vi "原始记录路径.vi"(9 "目标温度":string(combo), 11 "文件夹名称":string) -> (1 "file exists?":bool caption="文件或文件夹存在？", 3 "保存路径":path)   [LabVIEW 2015]
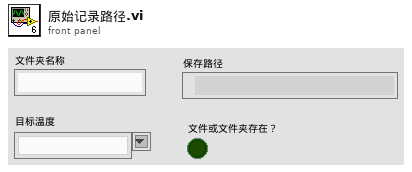
[diagram p1: front panel]
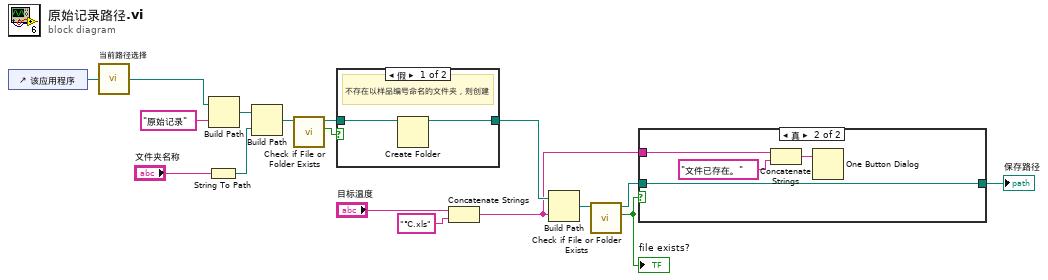
[diagram p0: block diagram]
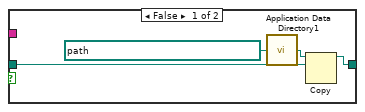
[diagram p2: hidden frame]
diagram:
  n1 = control-ref of="该应用程序"() -> (w17:refnum<vi>)
  n2 = call "当前路径选择.vi"("本应用程序"=w17) -> ("当前路径"=w16:path)
  n3 = String To Path(string="文件夹名称") -> (path=w1:path)
  n4 = Build Path(base path=w16, name or relative path="原始记录" ("名称或相对路径")) -> (appended path=w14:path)
  n5 = Build Path(base path=w14, name or relative path=w1) -> (appended path=w13:path)
  n6 = call <vilib>:"Check if File or Folder Exists.vi"("path"=w13) -> ("file or folder exists?"=w12:bool, "dup path"=w11:path)  [unwired: 8 in, 1 out]
  n7 = case shown="假" w12 {
    tunnel: w11 -> [w19 w20]
    tunnel: [w18 w20] -> w8
    frame False {
      # "不存在以样品编号命名的文件夹，则创建"
      n8 = Create Folder(path (use dialog)=w19) -> (created path=w18:path)  [unwired: 2 in, 2 out]
    }
    frame True {
    }
  }
  n9 = Concatenate Strings("目标温度", "℃.xls" ("字符串")) -> (w5:string)
  n10 = Build Path(base path=w8, name or relative path=w5) -> (appended path=w7:path)
  n11 = call <vilib>:"Check if File or Folder Exists.vi"("path"=w7) -> ("file or folder exists?"=w6:bool, "dup path"=w4:path)  [unwired: 8 in, 1 out]
  "file exists?" <- w6
  n12 = case shown="真" w6 {
    tunnel: w5 -> [_ w28]
    tunnel: w4 -> [w22 w25]
    tunnel: [w21 w25] -> w3
    frame False {
      n13 = call "Application Data Directory1.vi"("Relative path (.)"=path "恒温槽校准原始记录模板(公开).xls") -> ("Application Directory (+ Relative)"=w24:path)
      n14 = Copy(10:w22, 11:w24) -> (3:w21:path)  [unwired: 3 in, 2 out]
    }
    frame True {
      n15 = Concatenate Strings(w28, "文件已存在。" ("字符串")) -> (w26:string)
      n16 = One Button Dialog(message=w26) -> ()  [unwired: 1 in, 1 out]
    }
  }
  "保存路径" <- w3
